vi "Manual.vi"(0 "Right X":bool, 1 "Left X":bool, 2 "Up Y":bool, 3 "Down Y":bool, 4 "Out Z":bool, 5 "In Z":bool) -> (14 "EnviarSerial":string, 15 "Direccion":string)   [LabVIEW 2021]
panel:
  out "Contador":i32
  out "number":u32
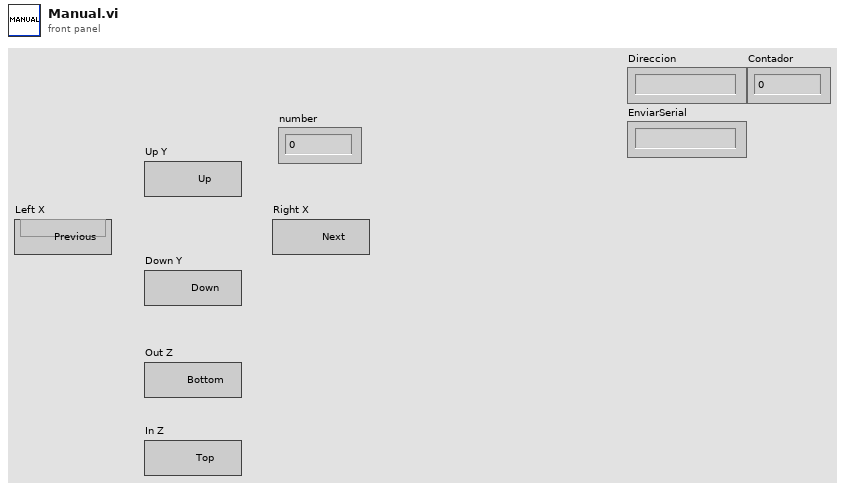
[diagram p1: front panel]
types:
  T1 = cluster{"Right X":bool, "Left X":bool, "Up Y":bool, "Down Y":bool, "In Z":bool, "Out Z":bool}
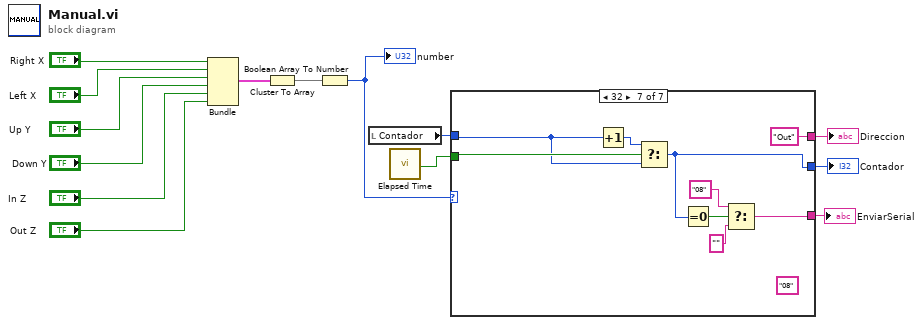
[diagram p0: block diagram]
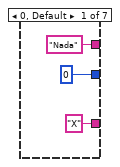
[diagram p2: hidden frame]
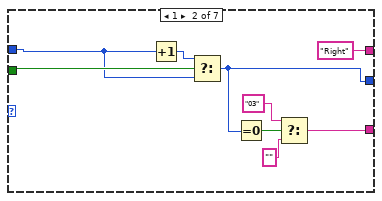
[diagram p3: hidden frame]
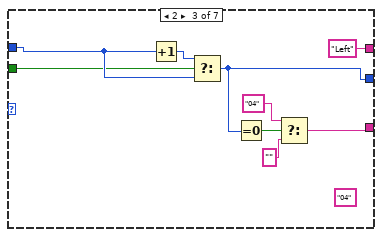
[diagram p4: hidden frame]
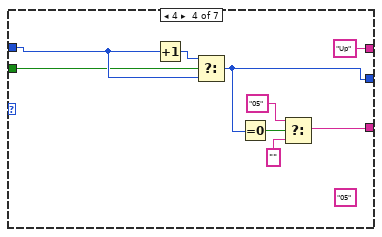
[diagram p5: hidden frame]
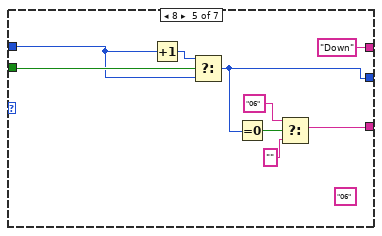
[diagram p6: hidden frame]
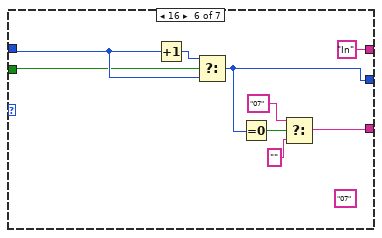
[diagram p7: hidden frame]
diagram:
  n1 = Bundle("Right X"="Right X", "Left X"="Left X", "Up Y"="Up Y", "Down Y"="Down Y", "In Z"="In Z", "Out Z"="Out Z") -> (w8:T1)  [unwired: 1 in]
  n2 = Cluster To Array(cluster=w8) -> (array=w7:bool[])
  n3 = Boolean Array To Number(Boolean array=w7) -> (number=w6:u32)
  "number" <- w6
  n4 = local read "Contador"() -> (w2:i32)
  n5 = call "Elapsed Time"() -> ("Time has Elapsed"=w3:bool)  [unwired: 12 in, 7 out]
  n6 = case shown="32" w6 {
    tunnel: ["Nada" "Right" "Left" "Up" "Down" "In" "Out"] -> w5
    tunnel: [0 w18 w29 w38 w45 w54 w65] -> w4
    tunnel: w3 -> [_ w25 w27 w36 w47 w55 w64]
    tunnel: w2 -> [_ w23 w28 w37 w46 w56 w63]
    tunnel: ["X" ("f") w19 w30 w39 w48 w57 w66] -> w1
    frame 0, Default {
    }
    frame 1 {
      n7 = Increment(x=w23) -> (x+1=w24:i32)
      n8 = Select(t=w24, s=w25, f=w23) -> (s? t:f=w18:i32)
      n9 = Equal To 0?(x=w18) -> (x = 0?=w22:bool)
      n10 = Select(t="03", s=w22, f="") -> (s? t:f=w19:string)
    }
    frame 2 {
      (unwired) "04"
      n11 = Increment(x=w28) -> (x+1=w34:i32)
      n12 = Select(t=w34, s=w27, f=w28) -> (s? t:f=w29:i32)
      n13 = Equal To 0?(x=w29) -> (x = 0?=w33:bool)
      n14 = Select(t="04", s=w33, f="") -> (s? t:f=w30:string)
    }
    frame 4 {
      (unwired) "05"
      n15 = Increment(x=w37) -> (x+1=w42:i32)
      n16 = Select(t=w42, s=w36, f=w37) -> (s? t:f=w38:i32)
      n17 = Equal To 0?(x=w38) -> (x = 0?=w43:bool)
      n18 = Select(t="05", s=w43, f="") -> (s? t:f=w39:string)
    }
    frame 8 {
      (unwired) "06"
      n19 = Increment(x=w46) -> (x+1=w52:i32)
      n20 = Select(t=w52, s=w47, f=w46) -> (s? t:f=w45:i32)
      n21 = Equal To 0?(x=w45) -> (x = 0?=w51:bool)
      n22 = Select(t="06", s=w51, f="") -> (s? t:f=w48:string)
    }
    frame 16 {
      (unwired) "07"
      n23 = Increment(x=w56) -> (x+1=w61:i32)
      n24 = Select(t=w61, s=w55, f=w56) -> (s? t:f=w54:i32)
      n25 = Equal To 0?(x=w54) -> (x = 0?=w60:bool)
      n26 = Select(t="07", s=w60, f="") -> (s? t:f=w57:string)
    }
    frame 32 {
      (unwired) "08"
      n27 = Increment(x=w63) -> (x+1=w70:i32)
      n28 = Select(t=w70, s=w64, f=w63) -> (s? t:f=w65:i32)
      n29 = Equal To 0?(x=w65) -> (x = 0?=w69:bool)
      n30 = Select(t="08", s=w69, f="") -> (s? t:f=w66:string)
    }
  }
  "Direccion" <- w5
  "EnviarSerial" <- w1
  "Contador" <- w4
